vi "Update_all_channels.vi"(11 "Channel Values":bool[][](array[boolean])) -> ()   [LabVIEW 2016]
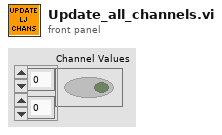
[diagram p1: front panel]
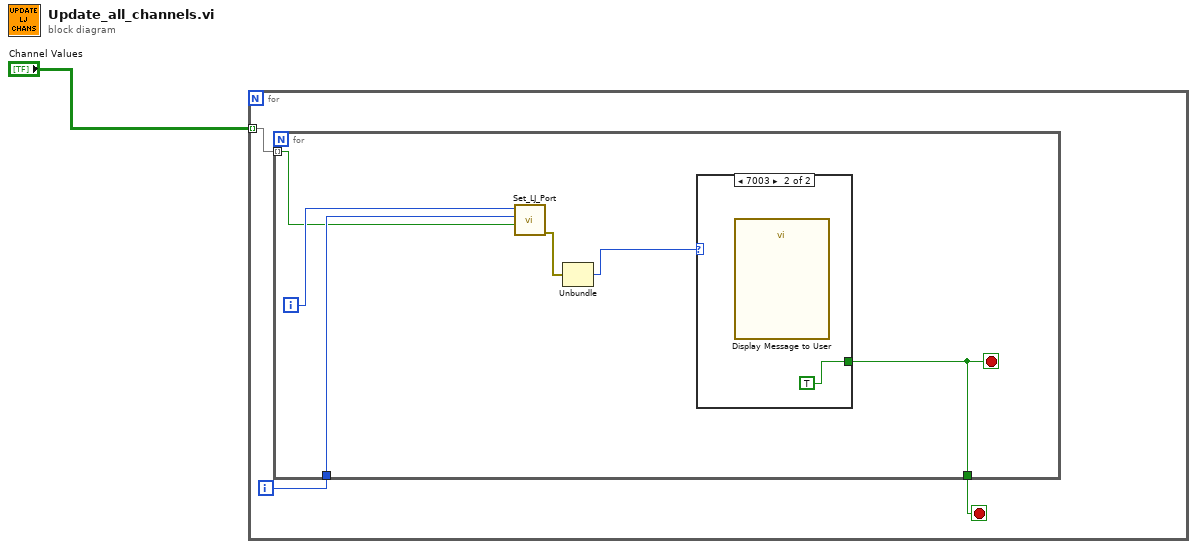
[diagram p0: block diagram]
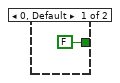
[diagram p2: hidden frame]
diagram:
  n1 = for {
    tunnel: "Channel Values" -> [w4] mode=indexing
    i -> [w3]
    stop <- w2 stop-if-true
    n2 = for {
      tunnel: w4 -> [w8] mode=indexing
      tunnel: w3 -> [w10]
      tunnel: [w5] -> w2
      i -> [w9]
      stop <- w5 stop-if-true
      n3 = call "Set_LJ_Port.vi"("State"=w8, "Channel"=w10, "Flowboard"=w9) -> ("error out"=w7:errorcluster)  [unwired: 8 in]
      n4 = Unbundle(w7) -> ("code"=w6:i32)  [unwired: 2 out]
      n5 = case shown="7003" w6 {
        tunnel: [FALSE TRUE] -> w5
        frame 0, Default {
        }
        frame 7003 {
          n6 = call "Display Message to User"() -> ()  [unwired: 10 in, 2 out]
        }
      }
    }
  }
